vi "GenRT_DebugOutput.vi"(2 "Line number ID":string, 4 "OutRefIdx for first node":i32=-1, 5 "prefix":string, 6 "Data ID":string, 7 "Variable Name ID":string, 8 "CodeParam in":refnum<class "CodeParam.lvclass">, 9 "error in (no error) ID":string, 10 "Type":refnum<class "Type.lvclass">, 11 "app ref":refnum<vi>) -> (0 "CodeParam out":refnum<class "CodeParam.lvclass">, 1 "error out ID":string, 3 "XML":string)   [LabVIEW 2021]
uses:
  <vilib>/imath/engines/lvmath2/MathScriptCompiler/Type.llb/Type.lvclass
  <vilib>/imath/engines/lvmath2/MathScriptCompiler/CodeParam.llb/CodeParam.lvclass
  <vilib>/imath/engines/lvmath2/Utility/RunTimeEnginePaths.ctl
  <vilib>/imath/engines/lvmath2/MathScriptCompiler/Code/XML Script.llb/XML Script - Cast Type To Target RunTimeType.vi
  <vilib>/imath/engines/lvmath2/MathScriptCompiler/Type/RuntimeType.llb/RuntimeType.lvclass
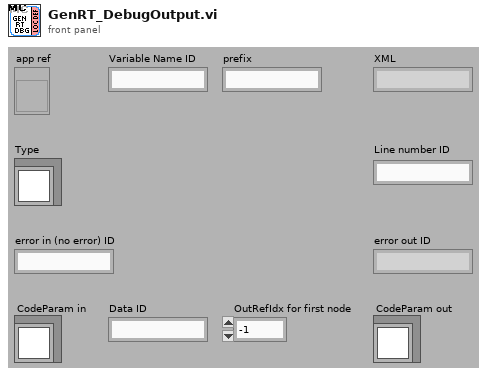
[diagram p1: front panel]
types:
  T1 = typedef "RunTimeEnginePaths.ctl" = u16
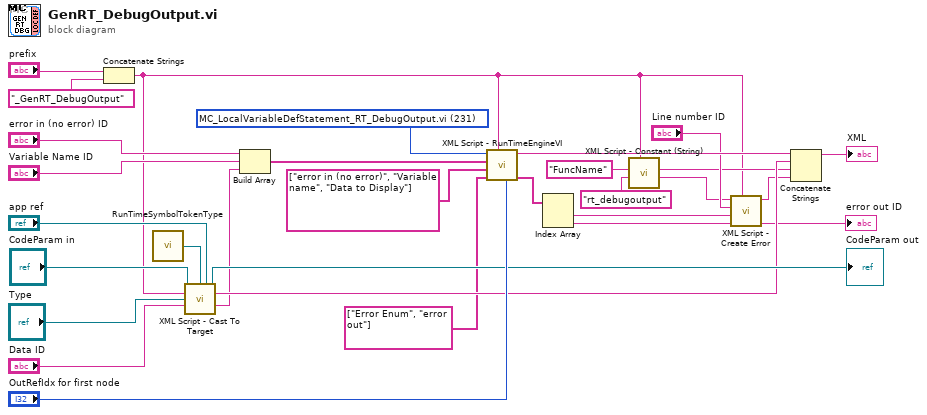
[diagram p0: block diagram]
diagram:
  w12 = T1 231 items=["You may add additional paths to the large string constant in 'GetRunTimeEnginePath.vi', but make sure to update 'RunTimeEnginePaths.ctl' and update the default value for the array as well", "NIMS_ArithmeticOperator_leftdiv.vi", "NIMS_ArithmeticOperator_minus.vi", "NIMS_ArithmeticOperator_leftdivmx.vi", "NIMS_ArithmeticOperator_powermx(M,M).vi", "NIMS_ArithmeticOperator_rightdivmx.vi", "NIMS_ArithmeticOperator_multmx.vi", "NIMS_ArithmeticOperator_plus.vi", "NIMS_power(GA,GA).vi", "NIMS_ArithmeticOperator_rightdiv.vi", "NIMS_ArithmeticOperator_times.vi", "NIMS_Bitwise_Operator_And.vi", "MC_Bitwise_Operator_Not.vi", "NIMS_Bitwise_Operator_Or.vi", "MC_BuiltInFunction_Invoke.vi", "MC_CommandStatement_break.vi", "MC_CommandStatement_return.vi", "MC_ForEndStatement_ Index Columns.vi", "MC_ForStatement_Get Iterations.vi", "MC_IfEndStatement_SelectCase.vi", "MC_LastElement_SymbolEnd.vi", "MC_LastElement_VariableEnd.vi", "MC_LocalVariableDefStatement_Ans.vi", "MC_LocalVariableDefStatement_Display.vi", "MC_Logical_Operator.vi", "UID Generator.vi", "MC_MatrixToken_Vertcat.vi", "MC_NodeBeginStatement_Init.vi", "MC_NodeEndStatement_Dispose.vi", "MC_OverloadedArithmeticOperator_Invoke.vi", "MC_Version.vi", "NIMS_Range.vi", "NIMS_Relational_Operator_Eq.vi", "NIMS_Relational_Operator_Ge.vi", "NIMS_Relational_Operator_Gt.vi", "NIMS_Relational_Operator_Le.vi", "NIMS_Relational_Operator_Lt.vi", "NIMS_Relational_Operator_Ne.vi", "MC_ReplaceToken_MC,MC,MC,MC.vi", "MC_ReplaceToken_MC,MC,MC.vi", "MC_ReplaceToken_MC,MC,x,MC.vi", "MC_ReplaceToken_MC,x,MC,MC.vi", "MC_ReplaceToken_MC,x,MC.vi", "MC_ReplaceToken_MC,x,x,MC.vi", "MC_ReplaceToken_MergeChildErrors.vi", "MC_RowToken_Horzcat.vi", "MC_SymbolToken_Invoke.vi", "MathScriptCompiler_VariableDefinition.vi", "MC_VariableToken_MC,MC,MC.vi", "MC_VariableToken_MC,MC,x.vi", "MC_VariableToken_MC,MC.vi", "MC_VariableToken_MC,x,MC.vi", "MC_VariableToken_MC,x.vi", "MC_VariableToken_VariableUse.vi", "MC_Mask_Errors.vi", "MC_CommandStatement_continue.vi", "MC_pi.vi", "MC_SwitchRelational_Operator_Eq.vi", "NIMS_ArithmeticOperator_multmx-internal.vi", "NIMS_Get Scalar - Matrix.vi", "NIMS_Get Row Vector - Matrix.vi", "NIMS_Get Column Vector - Matrix.vi", "NIMS_ArithmeticOperator_leftdivmx-internal.vi", "NIMS_ArithmeticOperator_rightdivmx-internal.vi", "NIMS_Get Scalar_w Error.vi", "NIMS_Get Row Vector_w Error - Matrix.vi", "NIMS_Get Column Vector_w Error - Matrix.vi", "NIMS_Complex To Real.vi", "NIMS_Get Any Vector_w Error - Matrix.vi", "NIMS_Error if Not Equal.vi", "NIMS_VariableToken_CondDefined.vi", "NIMS_NodeEndStatement_Output.vi", "NIMS_RowToken_CV_CV.vi", "NIMS_RowToken_CV_M.vi", "NIMS_RowToken_CV_SorRV.vi", "NIMS_RowToken_M_CV.vi", "NIMS_RowToken_M_M.vi", "NIMS_RowToken_M_SorRV.vi", "NIMS_RowToken_SorRV_CV.vi", "NIMS_RowToken_SorRV_M.vi", "NIMS_MatrixToken_M_M.vi", "NIMS_MatrixToken_M_RV.vi", "NIMS_MatrixToken_M_SorCV.vi", "NIMS_MatrixToken_RV_M.vi", "NIMS_MatrixToken_RV_RV.vi", "NIMS_MatrixToken_RV_SorCV.vi", "NIMS_MatrixToken_SorCV_M.vi", "NIMS_MatrixToken_SorCV_RV.vi", "NIMS_CH_String CV to Character 2D.vi", "NIMS_CH_Character 2D to String 2D.vi", "NIMS_CH_Character 2D to String 1D.vi", "NIMS_String to Enum.vi", "NIMS_Get Elements - _($) - safe.vi", "NIMS_Get Elements - _(_) - safe.vi", "NIMS_Get Elements - _(_,_) - safe.vi", "NIMS_Get Elements - _($,$) - safe.vi", "NIMS_Get Elements - _($,_) - safe.vi", "NIMS_Get Elements - _(_,$) - safe.vi", "NIMS_Get Elements - RowVector($,_) - safe.vi", "NIMS_Get Elements - ColumnVector($,_) - safe.vi", "NIMS_Get Elements - RowVector(_,$) - safe.vi", "NIMS_Get Elements - ColumnVector(_,$) - safe.vi", "NIMS_ArithmeticOperator_power(S).vi", "Write Variable.vi", "Read Variable.vi", "NIMS_RunTimeType To BaseType.vi", "NIMS_CH_String to Character Array.vi", "NIMS_CH_Character RV to String.vi", "NIMS_U8 2D to String 1D.vi", "NIMS_CH_Character 1D to U8 1D.vi", "NIMS_CH_Character 2D to U8 2D.vi", "Read UID Output Enabled.vi", "MC_Symbol_Table_Public_Read_TopLevelCallerUID.vi", "NIMS_RunTimeType_Get Case Value.vi", "NIMS_RunTimeType_To Numeric.vi", "NIMS_RunTimeType_From StrictType (excl LVString).vi", "NIMS_CH_U8 1D to Character 1D.vi", "NIMS_CH_U8 2D to Character 2D.vi", "Clear UID.vi", "NIMS_VariableToken_CondDefinedDefinedByReplace.vi", "NIMS_RunTimeSymbolToken_UserFunctionInvoke.vi", "NIMS_Compare Aggregates.vi", "NIMS_RunTimeSymbolToken_BuiltInFuncWrapperTemplate_1_1.vi", "NIMS_RunTimeSymbolToken_BuiltInFuncWrapperTemplate_2_1.vi", "NIMS_RunTimeSymbolToken_BuiltInFuncWrapperTemplate_2_2.vi", "NIMS_Get Elements - _(_,_) - nonstatic.vi", "NIMS_CD_Get Elements - _(_,_) - nonstatic.vi", "NIMS_Get Elements - _(_) - nonstatic.vi", "NIMS_CD_Get Elements - _(_) - nonstatic.vi", "NIMS_Get Elements - _($) - nonstatic.vi", "NIMS_CD_Get Elements - _($) - nonstatic.vi", "NIMS_Get Elements - _($,_) - nonstatic.vi", "NIMS_CD_Get Elements - _($,_) - nonstatic.vi", "NIMS_Get Elements - _(_,$) - nonstatic.vi", "NIMS_CD_Get Elements - _(_,$) - nonstatic.vi", "NIMS_Get Elements - _($,$) - nonstatic.vi", "NIMS_CD_Get Elements - _($,$) - nonstatic.vi", "NIMS_RowToken-nonstatic.vi", "NIMS_CD_RowToken-nonstatic.vi", "NIMS_MatrixToken-nonstatic.vi", "NIMS_CD_MatrixToken-nonstatic.vi", "NIMS_Finalize Error.vi", "NIMS_NodeEndStatement_Get Scalar.vi", "NIMS_NodeEndStatement_Get Vector.vi", "NIMS_BuiltInConstantToken_GetDims.vi", "NIMS_RuntimeSymbolToken_ReadVariable.vi", "Merge Error Enums.vi", "Matrix To Array - RM.vi", "Matrix To Array - CM.vi", "Array To Matrix - RA2.vi", "Array To Matrix - CA2.vi", "NIMS_RunTimeSymbolToken_Variant To 2D CDB.vi", "NIMS_RunTimeSymbolToken_Variant To 2D Char.vi", "NIMS_RunTimeSymbolToken_Variant To 2D Plot Object.vi", "NIMS_RunTimeSymbolToken_Variant To 2D ZPK Object.vi", "NIMS_RunTimeSymbolToken_Variant To 2D SS Object.vi", "NIMS_RunTimeSymbolToken_Variant To 2D TF Object.vi", "NIMS_Clear Errors.vi", "NIMS_RuntimeSymbolToken_ResolveSymbol.vi", "NIMS_CD_RunTimeSymbolToken_ResolveSymbol.vi", "NIMS_NS_ArithmeticOperator_cctranspose.vi", "NIMS_NS_ArithmeticOperator_leftdiv.vi", "NIMS_NS_ArithmeticOperator_leftdivmx.vi", "NIMS_NS_ArithmeticOperator_minus.vi", "NIMS_NS_ArithmeticOperator_multmx.vi", "NIMS_NS_ArithmeticOperator_plus.vi", "NIMS_NS_ArithmeticOperator_power.vi", "NIMS_NS_ArithmeticOperator_powermx.vi", "NIMS_NS_ArithmeticOperator_rightdiv.vi", "NIMS_NS_ArithmeticOperator_rightdivmx.vi", "NIMS_NS_ArithmeticOperator_times.vi", "NIMS_NS_ArithmeticOperator_transpose.vi", "NIMS_CD_NS_ArithmeticOperator_plus.vi", "NIMS_CD_NS_ArithmeticOperator_minus.vi", "NIMS_CD_NS_ArithmeticOperator_multmx.vi", "NIMS_CD_NS_ArithmeticOperator_leftdivmx.vi", "NIMS_CD_NS_ArithmeticOperator_rightdivmx.vi", "NIMS_CD_NS_ArithmeticOperator_powermx.vi", "NIMS_CD_NS_ArithmeticOperator_cctranspose.vi", "NIMS_NS_Relational_Operator_Eq.vi", "NIMS_NS_Relational_Operator_Lt.vi", "NIMS_NS_Relational_Operator_Gt.vi", "NIMS_NS_Relational_Operator_Le.vi", "NIMS_NS_Relational_Operator_Ge.vi", "NIMS_NS_Relational_Operator_Ne.vi", "NIMS_NS_Bitwise_Operator_And.vi", "NIMS_NS_Bitwise_Operator_Or.vi", "NIMS_NS_Bitwise_Operator_Not.vi", "NIMS_NS_Range - 2 inputs.vi", "NIMS_NS_Range - 3 inputs.vi", "NIMS_RunTimeSymbolToken_ResolveUDForVariable.vi", "NIMS_CD_RunTimeSymbolToken_ResolveUDForVariable.vi", "NIMS_ArithmeticOperator_leftdiv(C,C).vi", "NIMS_ArithmeticOperator_leftdivmx(C,C).vi", "NIMS_ArithmeticOperator_rightdiv(C,C).vi", "NIMS_ArithmeticOperator_rightdivmx(C,C).vi", "NIMS_ArithmeticOperator_rightdivmx(C,C)-internal.vi", "NIMS_ArithmeticOperator_leftdivmx(C,C)-internal.vi", "NIMS_CD_NS_LoopVariableIndexToken_Index.vi", "NIMS_NS_LoopVariableIndexToken_Index.vi", "NIMS_NS_LastElementToken_First.vi", "NIMS_NS_LastElementToken_Second.vi", "NIMS_NS_LastElementToken_Only.vi", "NIMS_CD_NS_LastElementToken_First.vi", "NIMS_CD_NS_LastElementToken_Second.vi", "NIMS_CD_NS_LastElementToken_Only.vi", "NIMS_NS_Replace - M($)=M.vi", "NIMS_NS_Replace - M(M)=M.vi", "NIMS_NS_Replace - M($,$)=M.vi", "NIMS_NS_Replace - M($,M)=M.vi", "NIMS_NS_Replace - M(M,$)=M.vi", "NIMS_NS_Replace - M(M,M)=M.vi", "NIMS_Range_R2.vi", "NIMS_Range_R3.vi", "NIMS_CommandStatement_MaskErr.vi", "NIMS_Range_R2 - Integer.vi", "NIMS_Range_R3 - Integer.vi", "NIMS_Range_R2 - Float.vi", "NIMS_Range_R3 - Float.vi", "NIMS_UserFunction_CondDefined.vi", "MC_Error Cluster From Error Code.vi", "MC_Mask_Errors.vi", "MergeErrorsWrapper.vi", "Initialize Plug In List.vi", "Create Error.vi", "NIMS_ArithmeticOperator_multmx(M,CV).vi", "NIMS_ArithmeticOperator_multmx(M,CV)-internal.vi", "NIMS_ArithmeticOperator_multmx(RV,M).vi", "NIMS_ArithmeticOperator_multmx(RV,M)-internal.vi", "NIMS_ArithmeticOperator_multmx(RV,CV).vi", "NIMS_ArithmeticOperator_multmx(RV,CV)-internal.vi", "MC_LocalVariableDefStatement_RT_DebugOutput.vi"] ("RunTimeEngine VI")
  n1 = Concatenate Strings("prefix", "_GenRT_DebugOutput" ("string")) -> (w1:string)
  n2 = call <vilib>:"RunTimeSymbolTokenType.vi"() -> ("RunTimeSymbolTokenType"=w18:refnum<class "RuntimeType.lvclass">)  [unwired: 1 out]
  n3 = call-poly <vilib>:"XML Script - Cast To Target.vi"("CodeParam in"="CodeParam in", "Target RunTimeType"=w18, "app ref"="app ref", "prefix"=w1, "Type"="Type", "Term ID (in)"="Data ID") -> ("CodeParam out"=→"CodeParam out":refnum<class "CodeParam.lvclass">, "XML"=w17:string, "Term ID (out)"=w16:string)  [unwired: 1 in, 6 out]
  n4 = Build Array("error in (no error) ID", "Variable Name ID", w16) -> (w14:string[])
  n5 = call <vilib>:"XML Script - RunTimeEngineVI.vi"("out"="OutRefIdx for first node", "prefix"=w1, "Output Term Names"=string[] ["Error Enum", "error out"], "Input Term Names"=string[] ["error in (no error)", "Variable name", "Data to Display"], "Input TermIDs"=w14, "RunTimeEngine VI"=w12) -> ("Output TermIDs"=w15:string[], "XML"=w19:string)  [unwired: 4 out]
  n6 = Index Array(array=w15) -> (element #1=w10:string, element #2=w9:string)  [unwired: 2 in]
  n7 = call <vilib>:"XML Script - Constant (String).vi"("value"="rt_debugoutput", "name"="FuncName", "prefix (name)"=w1) -> ("name (wire source)"=w4:string, "XML Script Command - Constant (I32)"=w2:string)  [unwired: 4 in, 3 out]
  n8 = call <vilib>:"XML Script - Create Error.vi"("prefix (name)"=w1, "error in (no error) ID"=w9, "Error Enum ID"=w10, "Line number ID"="Line number ID", "Function name ID"=w4) -> ("error out ID"=→"error out ID":string, "XML"=w3:string)  [unwired: 5 in]
  n9 = Concatenate Strings(w19, w17, w2, w3) -> (→"XML":string)
